vi "rp_change_representation.vi"(6 "Variant in":variant, 7 "Shift Pressed?":bool, 8 "error in (no error)":errorcluster, 10 "QD Combo Box Ref":refnum<vi>, 11 "QD Launch VI Ref":refnum<vi>) -> (0 "error out":errorcluster, 4 "Variant out":variant)   [LabVIEW 2019]
doc: "Change the selected numeric or string control/constant representation, radix and modifiers using the quick drop combo box text formatted as: \"[TYPE[ MODS...]]\"\nTYPE = 'u8', 'u16', 'u32', 'u64', 'i8', 'i16', 'i32', 'i64', 'sgl', 'dbl', 'ext'\nMODS = \n 'd': dec/default\n 'x': hex\n 'b': bin/backslash\n 'r': toggle radix visible\n 'h': hide inc/dec buttons\n 's': show inc/dec buttons\n\nExamples:\nNumeric selected +\"u8 x h\" = Unsigned 8-bit representation, display radix as hex and hide inc/dec buttons\nString selected + \"b\" = Display radix in backslash\n\nDefault Shortcut - [V]"
uses:
  <vilib>/numeric/LVNumericRepresentation.ctl
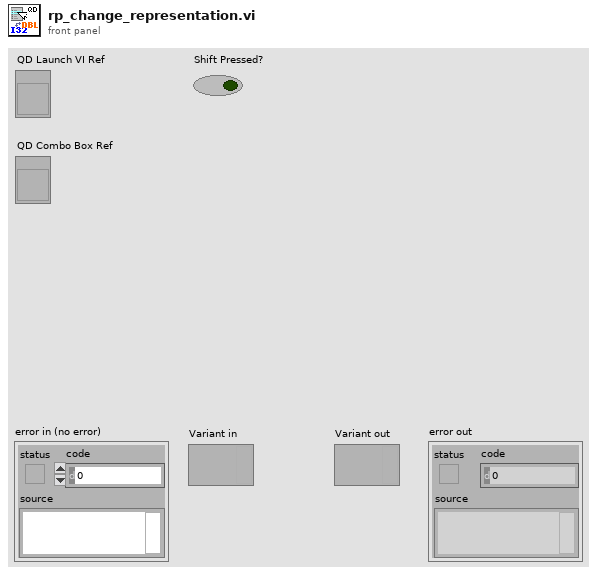
[diagram p1: front panel]
types:
  T1 = typedef "LVNumericRepresentation.ctl" = enum32{"Extended Precision", "Double Precision", "Single Precision", "Long", "Word", "Byte", "Unsigned Long", "Unsigned Word", "Unsigned Byte", "Complex Extended", "Complex Double", "Complex Single", "Quad", "Unsigned Quad", "Fixed-Point"}
  T2 = enum8{"none", "toggle", "decimal", "hex", "binary"}
  T3 = cluster{"DigitalCst":refnum<vi>[], "EnumCst":refnum<vi>[], "RingCst":refnum<vi>[], "StringCst":refnum<vi>[], "Digitals":refnum<vi>[], "Enums":refnum<vi>[], "Rings":refnum<vi>[], "Strings":refnum<vi>[]}
  T4 = typedef "LVRectTypeDef.ctl" = cluster{"Left":i16, "Top":i16, "Right":i16, "Bottom":i16}
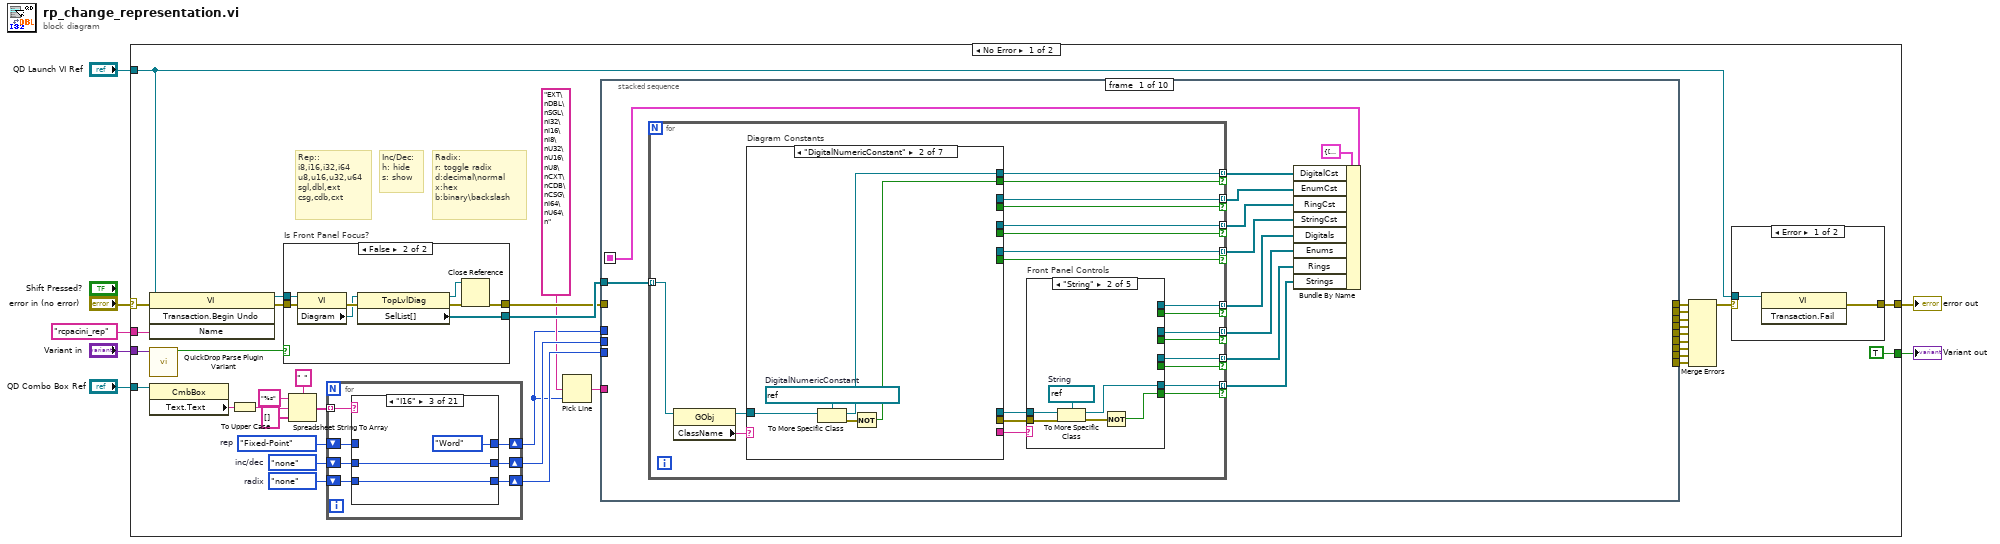
[diagram p0: block diagram]
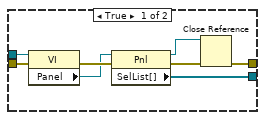
[diagram p2: hidden frame]
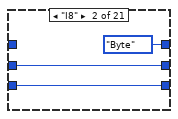
[diagram p4: hidden frame]
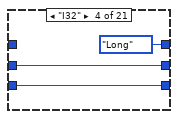
[diagram p5: hidden frame]
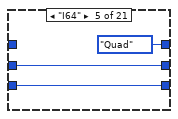
[diagram p6: hidden frame]
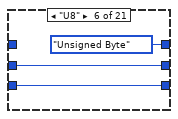
[diagram p7: hidden frame]
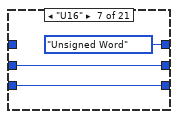
[diagram p8: hidden frame]
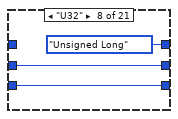
[diagram p9: hidden frame]
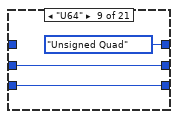
[diagram p10: hidden frame]
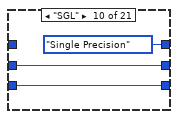
[diagram p11: hidden frame]
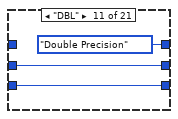
[diagram p12: hidden frame]
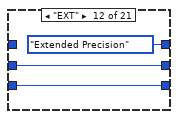
[diagram p13: hidden frame]
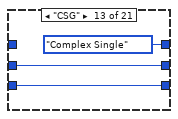
[diagram p14: hidden frame]
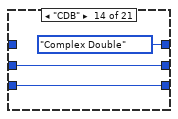
[diagram p15: hidden frame]
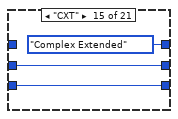
[diagram p16: hidden frame]
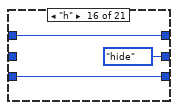
[diagram p17: hidden frame]
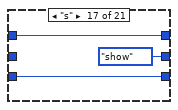
[diagram p18: hidden frame]
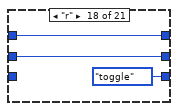
[diagram p19: hidden frame]
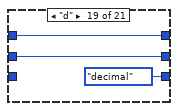
[diagram p20: hidden frame]
diagram:
  n1 = case shown="No Error" "error in (no error)" {
    selector: "error in (no error)" -> [w43 w671]
    tunnel: [w42 w671] -> w1
    tunnel: "QD Launch VI Ref" -> [w36 _]
    tunnel: "rcpacini_rep" ("Undo Name") -> [w41 _]
    tunnel: "Variant in" -> [w9 _]
    tunnel: "QD Combo Box Ref" -> [w37 _]
    tunnel: [TRUE _] -> w2
    frame No Error {
      w26 = enum8{"none", "show", "hide"}."none"  # inc/dec
      w27 = T2."none"  # radix
      w28 = LVNumericRepresentation."Fixed-Point"  # rep
      # "Radix:\nr: toggle radix\nd:decimal\\normal\nx:hex\nb:binary\\backslash"
      # "Inc/Dec:\nh: hide\ns: show"
      # "Rep::\ni8,i16,i32,i64\nu8,u16,u32,u64\nsgl,dbl,ext\ncsg,cdb,cxt"
      n2 = invoke class="VI" method="Transaction.Begin Undo"(reference=w36, error in=w43, "Name"=w41) -> (reference out=w39:refnum<vi>, error out=w40:errorcluster)  [unwired: 1 in, 2 out]
      n3 = call <vilib>:"QuickDrop Parse Plugin Variant.vi"("QDKS Variant in"=w9) -> ("QD Launch VI Panel?"=w8:bool)  [unwired: 12 in, 2 out]
      n4 = property class="CmbBox"(reference=w37) -> ("Text.Text"=w35:string)  [unwired: 1 in, 2 out]
      n5 = To Upper Case(1:w35) -> (0:w34:string)
      n6 = case "Is Front Panel Focus?" shown="False" w8 {
        tunnel: w40 -> [w51 w59]
        tunnel: w39 -> [w50 w58]
        tunnel: [w45 w53] -> w25
        tunnel: [w44 w52] -> w30
        frame True {
          n7 = property class="VI"(reference=w50, error in=w51) -> (error out=w49:errorcluster, "Panel"=w48:refnum<vi>)  [unwired: 1 out]
          n8 = property class="Pnl"(reference=w48, error in=w49) -> (reference out=w46:refnum<vi>, error out=w47:errorcluster, "SelList[]"=w44:refnum<vi>[])
          n9 = Close Reference(reference=w46, error in (no error)=w47) -> (error out=w45:errorcluster)
        }
        frame False {
          n10 = property class="VI"(reference=w58, error in=w59) -> (error out=w57:errorcluster, "Diagram"=w56:refnum<vi>)  [unwired: 1 out]
          n11 = property class="TopLvlDiag"(reference=w56, error in=w57) -> (reference out=w54:refnum<vi>, error out=w55:errorcluster, "SelList[]"=w52:refnum<vi>[])
          n12 = Close Reference(reference=w54, error in (no error)=w55) -> (error out=w53:errorcluster)
        }
      }
      n13 = Spreadsheet String To Array(delimiter (Tab)=" ", format string="%s", spreadsheet string=w34, array type (2D Dbl)=string[] []) -> (array=w29:string[])
      n14 = for {
        tunnel: w29 -> [w66] mode=indexing
        shift-right: [w64] -> w11
        shift-left: w28 -> [w65]
        shift-right: [w63] -> w23
        shift-left: w26 -> [w62]
        shift-right: [w60] -> w22
        shift-left: w27 -> [w61]
        n15 = case shown="\"I16\"" w66 {
          tunnel: w65 -> [w69 _ _ _ _ _ _ _ _ _ _ _ _ _ _ w114 w117 w120 w123 w126 w129]
          tunnel: [w69 LVNumericRepresentation."Byte" ("Representation") LVNumericRepresentation."Word" ("Representation") LVNumericRepresentation."Long" ("Representation") LVNumericRepresentation."Quad" ("Representation") LVNumericRepresentation."Unsigned Byte" ("Representation") LVNumericRepresentation."Unsigned Word" ("Representation") LVNumericRepresentation."Unsigned Long" ("Representation") LVNumericRepresentation."Unsigned Quad" ("Representation") LVNumericRepresentation."Single Precision" ("Representation") LVNumericRepresentation."Double Precision" ("Representation") LVNumericRepresentation."Extended Precision" ("Representation") LVNumericRepresentation."Complex Single" ("Representation") LVNumericRepresentation."Complex Double" ("Representation") LVNumericRepresentation."Complex Extended" ("Representation") w114 w117 w120 w123 w126 w129] -> w64
          tunnel: [w68 w71 w74 w77 w80 w83 w86 w89 w92 w95 w98 w101 w104 w107 w110 enum8{"none", "show", "hide"}."hide" ("inc/dec") enum8{"none", "show", "hide"}."show" ("inc/dec") w119 w122 w125 w128] -> w63
          tunnel: w62 -> [w68 w71 w74 w77 w80 w83 w86 w89 w92 w95 w98 w101 w104 w107 w110 _ _ w119 w122 w125 w128]
          tunnel: [w67 w70 w73 w76 w79 w82 w85 w88 w91 w94 w97 w100 w103 w106 w109 w113 w116 T2."toggle" ("radix") T2."decimal" ("radix") T2."hex" ("radix") T2."binary" ("radix")] -> w60
          tunnel: w61 -> [w67 w70 w73 w76 w79 w82 w85 w88 w91 w94 w97 w100 w103 w106 w109 w113 w116 _ _ _ _]
          frame Default {
          }
          frame "I8" {
          }
          frame "I16" {
          }
          frame "I32" {
          }
          frame "I64" {
          }
          frame "U8" {
          }
          frame "U16" {
          }
          frame "U32" {
          }
          frame "U64" {
          }
          frame "SGL" {
          }
          frame "DBL" {
          }
          frame "EXT" {
          }
          frame "CSG" {
          }
          frame "CDB" {
          }
          frame "CXT" {
          }
          frame "h" {
          }
          frame "s" {
          }
          frame "r" {
          }
          frame "d" {
          }
          frame "x" {
          }
          frame "b" {
          }
        }
      }
      n16 = Pick Line(multi-line string="EXT\nDBL\nSGL\nI32\nI16\nI8\nU32\nU16\nU8\nCXT\nCDB\nCSG\nI64\nU64\n", line index=w11) -> (output string=w10:string)  [unwired: 1 in]
      n17 = stacked-sequence {
        seq-local: [w130 _ _ _ _ _ _ _ _ _] -> [_ w220 w312 w350 w388 w438 w535 w574 w616 _]
        tunnel: w30 -> [w140 _ _ _ _ _ _ _ _ w666]
        tunnel: w25 -> [_ w219 w311 w349 w387 w437 w534 w573 w615 w665]
        tunnel: w11 -> [_ w224 w314 w352 _ w441 w537 w576 _ _]
        tunnel: w23 -> [_ w223 _ _ w389 w440 w536 w575 w617 _]
        tunnel: w22 -> [_ w222 _ _ w390 w439 _ _ w618 _]
        tunnel: [_ w218 _ _ _ _ _ _ _ _] -> w24
        tunnel: w10 -> [_ w221 w313 w351 _ _ _ _ _ _]
        tunnel: [_ _ w310 _ _ _ _ _ _ _] -> w21
        tunnel: [_ _ _ w348 _ _ _ _ _ _] -> w20
        tunnel: [_ _ _ _ w386 _ _ _ _ _] -> w19
        tunnel: [_ _ _ _ _ w436 _ _ _ _] -> w18
        tunnel: [_ _ _ _ _ _ w533 _ _ _] -> w17
        tunnel: [_ _ _ _ _ _ _ w572 _ _] -> w16
        tunnel: [_ _ _ _ _ _ _ _ w614 _] -> w15
        tunnel: [_ _ _ _ _ _ _ _ _ w664] -> w14
        frame #0 {
          n18 = for {
            tunnel: w140 -> [w162] mode=indexing
            tunnel: [w159] -> w139 mode=indexing if=w158
            tunnel: [w157] -> w138 mode=indexing if=w156
            tunnel: [w155] -> w137 mode=indexing if=w154
            tunnel: [w153] -> w136 mode=indexing if=w152
            tunnel: [w148] -> w132 mode=indexing if=w147
            tunnel: [w146] -> w135 mode=indexing if=w145
            tunnel: [w144] -> w134 mode=indexing if=w143
            tunnel: [w142] -> w133 mode=indexing if=w141
            n19 = property class="GObj"(reference=w162) -> (reference out=w160:refnum<vi>, "ClassName"=w161:string)  [unwired: 1 in, 1 out]
            n20 = case "Diagram Constants" shown="\"DigitalNumericConstant\"" w161 {
              selector: w161 -> [_ _ _ _ _ _ w216]
              tunnel: w160 -> [_ w190 w195 w200 w205 w214 w217]
              tunnel: [_ w189 _ _ _ _ _] -> w159
              tunnel: [_ w187 _ _ _ _ _] -> w158
              tunnel: [_ _ w193 _ _ _ _] -> w157
              tunnel: [_ _ w192 _ _ _ _] -> w156
              tunnel: [_ _ _ w198 _ _ _] -> w155
              tunnel: [_ _ _ w197 _ _ _] -> w154
              tunnel: [_ _ _ _ w203 _ _] -> w153
              tunnel: [_ _ _ _ w202 _ _] -> w152
              tunnel: [_ _ _ _ _ w209 w216] -> w149
              tunnel: [_ _ _ _ _ w208 w217] -> w151
              tunnel: [_ _ _ _ _ w207 _] -> w150
              frame Default {
              }
              frame "DigitalNumericConstant" {
                w191 = refnum<vi> refnum  # DigitalNumericConstant
                n21 = To More Specific Class(target class=w191, reference=w190) -> (specific class reference=w189:refnum<vi>, error out=w188:errorcluster)  [unwired: 1 in]
                n22 = Not(x=w188) -> (.not. x?=w187:bool)
              }
              frame "EnumConstant" {
                w196 = refnum<vi> refnum  # EnumConstant
                n23 = To More Specific Class(target class=w196, reference=w195) -> (specific class reference=w193:refnum<vi>, error out=w194:errorcluster)  [unwired: 1 in]
                n24 = Not(x=w194) -> (.not. x?=w192:bool)
              }
              frame "RingConstant" {
                w201 = refnum<vi> refnum  # RingConstant
                n25 = To More Specific Class(target class=w201, reference=w200) -> (specific class reference=w198:refnum<vi>, error out=w199:errorcluster)  [unwired: 1 in]
                n26 = Not(x=w199) -> (.not. x?=w197:bool)
              }
              frame "StringConstant" {
                w206 = refnum<vi> refnum  # StringConstant
                n27 = To More Specific Class(target class=w206, reference=w205) -> (specific class reference=w203:refnum<vi>, error out=w204:errorcluster)  [unwired: 1 in]
                n28 = Not(x=w204) -> (.not. x?=w202:bool)
              }
              frame "ControlTerminal" {
                w215 = refnum<vi> refnum  # ControlTerminal
                n29 = To More Specific Class(target class=w215, reference=w214) -> (specific class reference=w211:refnum<vi>, error out=w213:errorcluster)  [unwired: 1 in]
                n30 = property class="CtrlTerm"(reference=w211, error in=w213) -> (error out=w212:errorcluster, "Control"=w210:refnum<vi>)  [unwired: 1 out]
                n31 = property class="Ctl"(reference=w210, error in=w212) -> (reference out=w208:refnum<vi>, error out=w207:errorcluster, "ClassName"=w209:string)
              }
              frame "Digital", "Enum", "Ring", "String" {
              }
            }
            n32 = case "Front Panel Controls" shown="\"String\"" w149 {
              tunnel: w151 -> [_ w167 w173 w179 w185]
              tunnel: w150 -> [_ w166 w172 w178 w184]
              tunnel: [_ w164 _ _ _] -> w148
              tunnel: [_ w163 _ _ _] -> w147
              tunnel: [_ _ w170 _ _] -> w146
              tunnel: [_ _ w169 _ _] -> w145
              tunnel: [_ _ _ w176 _] -> w144
              tunnel: [_ _ _ w175 _] -> w143
              tunnel: [_ _ _ _ w182] -> w142
              tunnel: [_ _ _ _ w181] -> w141
              frame Default {
              }
              frame "String" {
                w168 = refnum<vi> refnum  # String
                n33 = To More Specific Class(target class=w168, reference=w167, error in=w166) -> (specific class reference=w164:refnum<vi>, error out=w165:errorcluster)
                n34 = Not(x=w165) -> (.not. x?=w163:bool)
              }
              frame "Digital" {
                w174 = refnum<vi> refnum  # Digital
                n35 = To More Specific Class(target class=w174, reference=w173, error in=w172) -> (specific class reference=w170:refnum<vi>, error out=w171:errorcluster)
                n36 = Not(x=w171) -> (.not. x?=w169:bool)
              }
              frame "Enum" {
                w180 = refnum<vi> refnum  # Enum
                n37 = To More Specific Class(target class=w180, reference=w179, error in=w178) -> (specific class reference=w176:refnum<vi>, error out=w177:errorcluster)
                n38 = Not(x=w177) -> (.not. x?=w175:bool)
              }
              frame "Ring" {
                w186 = refnum<vi> refnum  # Ring
                n39 = To More Specific Class(target class=w186, reference=w185, error in=w184) -> (specific class reference=w182:refnum<vi>, error out=w183:errorcluster)
                n40 = Not(x=w183) -> (.not. x?=w181:bool)
              }
            }
          }
          n41 = Bundle By Name(cluster=T3 {"DigitalCst"=[], "EnumCst"=[], "RingCst"=[], "StringCst"=[], "Digitals"=[], "Enums"=[], "Rings"=[], "Strings"=[]} ("refnums"), "DigitalCst"=w139, "EnumCst"=w138, "RingCst"=w137, "StringCst"=w136, "Digitals"=w135, "Enums"=w134, "Rings"=w133, "Strings"=w132) -> (w130:T3)
        }
        frame #1 {
          # "Digital Constants"
          n42 = Unbundle By Name(w220) -> ("DigitalCst"=w225:refnum<vi>[])
          n43 = for {
            tunnel: w225 -> [w238] mode=indexing
            tunnel: w224 -> [w236]
            tunnel: w223 -> [_]
            tunnel: w222 -> [w235]
            tunnel: w219 -> [w237]
            tunnel: w221 -> [w227]
            shift-right: [w229] -> w218
            shift-left: w219 -> [w228]
            n44 = case shown="Default" w236 {
              selector: w236 -> [_ w306]
              tunnel: w238 -> [w302 w309]
              tunnel: w237 -> [w303 w308]
              tunnel: [w303 w307] -> w231
              tunnel: [w302 w305] -> w230
              tunnel: [_ w304] -> w226
              tunnel: w227 -> [_ w304]
              frame "Fixed-Point" {
              }
              frame Default {
                n45 = property class="DigCnst"(reference=w309, error in=w308, "Representation"=w306) -> (reference out=w305:refnum<vi>, error out=w307:errorcluster)
              }
            }
            n46 = case shown="\"decimal\"" w235 {
              tunnel: w231 -> [w254 w260 w271 w285 w301]
              tunnel: w230 -> [w253 w258 w269 w283 w300]
              tunnel: [w254 w262 w273 w287 w296] -> w234
              tunnel: [w253 w261 w272 w286 w294] -> w232
              frame "none" {
              }
              frame "decimal" {
                n47 = property class="DigCnst"(reference=w258, error in=w260) -> (reference out=w257:refnum<vi>, error out=w259:errorcluster, "Representation"=w256:T1)
                n48 = case shown="\"Long\"..\"Unsigned Byte\", \"Quad\", \"Unsigned Quad\"" w256 {
                  tunnel: [_ "%d" "%#_13g"] -> w255
                  frame "Fixed-Point" {
                  }
                  frame "Long".."Unsigned Byte", "Quad", "Unsigned Quad" {
                  }
                  frame "Extended Precision".."Single Precision", "Complex Extended".."Complex Single" {
                  }
                }
                n49 = property class="DigCnst"(reference=w257, error in=w259, "RadixVis"=TRUE ("Radix Visible?"), "FormatString"=w255) -> (reference out=w261:refnum<vi>, error out=w262:errorcluster)
              }
              frame "hex" {
                n50 = property class="DigCnst"(reference=w269, error in=w271) -> (reference out=w268:refnum<vi>, error out=w270:errorcluster, "Representation"=w267:T1)
                n51 = case shown="\"Extended Precision\"..\"Single Precision\", \"Complex Extended\"..\"Complex Single\"" w267 {
                  tunnel: [_ "%02x" "%04x" "%08x" "%016x" "%#_13g"] -> w266
                  frame "Fixed-Point" {
                  }
                  frame "Byte", "Unsigned Byte" {
                  }
                  frame "Word", "Unsigned Word" {
                  }
                  frame "Long", "Unsigned Long" {
                  }
                  frame "Quad", "Unsigned Quad" {
                  }
                  frame "Extended Precision".."Single Precision", "Complex Extended".."Complex Single" {
                  }
                }
                n52 = property class="DigCnst"(reference=w268, error in=w270, "RadixVis"=TRUE ("Radix Visible?"), "FormatString"=w266) -> (reference out=w272:refnum<vi>, error out=w273:errorcluster)
              }
              frame "binary" {
                n53 = property class="DigCnst"(reference=w283, error in=w285) -> (reference out=w282:refnum<vi>, error out=w284:errorcluster, "Representation"=w280:T1)
                n54 = case shown="\"Byte\", \"Unsigned Byte\"" w280 {
                  tunnel: [_ "%08b" "%016b" "%032b" "%064b" "%#_13g"] -> w281
                  frame "Fixed-Point" {
                  }
                  frame "Byte", "Unsigned Byte" {
                  }
                  frame "Word", "Unsigned Word" {
                  }
                  frame "Long", "Unsigned Long" {
                  }
                  frame "Quad", "Unsigned Quad" {
                  }
                  frame "Extended Precision".."Single Precision", "Complex Extended".."Complex Single" {
                  }
                }
                n55 = property class="DigCnst"(reference=w282, error in=w284, "RadixVis"=TRUE ("Radix Visible?"), "FormatString"=w281) -> (reference out=w286:refnum<vi>, error out=w287:errorcluster)
              }
              frame "toggle" {
                n56 = property class="DigCnst"(reference=w300, error in=w301) -> (reference out=w298:refnum<vi>, error out=w299:errorcluster, "RadixVis"=w297:bool)
                n57 = Not(x=w297) -> (.not. x?=w295:bool)
                n58 = property class="DigCnst"(reference=w298, error in=w299, "RadixVis"=w295) -> (reference out=w294:refnum<vi>, error out=w296:errorcluster)
              }
            }
            n59 = case shown="Default" w226 {
              selector: w226 -> [_ w249]
              tunnel: w234 -> [w239 w252]
              tunnel: [w239 w241] -> w233
              tunnel: w232 -> [_ w251]
              frame "" {
              }
              frame Default {
                n60 = property class="DigCnst"(reference=w251, error in=w252, "Label.Visible"=TRUE, "Label.Text"=w249) -> (reference out=w247:refnum<vi>, error out=w248:errorcluster)
                n61 = property class="DigCnst"(reference=w247, error in=w248) -> (error out=w240:errorcluster, "Label"=w246:refnum<vi>, "MasterRect"=w244:T4)  [unwired: 1 out]
                n62 = call "rp_move_label.vi"("error in (no error)"=w240, "Master Bounds Rect"=w244, "Is Source? (F)"=TRUE, "Label in"=w246) -> ("error out"=w242:errorcluster, "dup Label"=w243:refnum<vi>)  [unwired: 6 in]
                n63 = Close Reference(reference=w243, error in (no error)=w242) -> (error out=w241:errorcluster)
              }
            }
            n64 = Merge Errors(w228, w233) -> (w229:errorcluster)
          }
        }
        frame #2 {
          # "Enum Constants"
          n65 = Unbundle By Name(w312) -> ("EnumCst"=w315:refnum<vi>[])
          n66 = for {
            tunnel: w315 -> [w325] mode=indexing
            tunnel: w314 -> [w323]
            tunnel: w311 -> [w324]
            tunnel: w313 -> [w316]
            shift-right: [w319] -> w310
            shift-left: w311 -> [w318]
            n67 = case shown="\"Unsigned Long\"..\"Unsigned Byte\"" w323 {
              selector: w323 -> [_ w344]
              tunnel: w325 -> [w340 w347]
              tunnel: w324 -> [w341 w346]
              tunnel: [w341 w345] -> w322
              tunnel: [w340 w343] -> w321
              tunnel: [_ w342] -> w317
              tunnel: w316 -> [_ w342]
              frame Default {
              }
              frame "Unsigned Long".."Unsigned Byte" {
                n68 = property class="EnmCnst"(reference=w347, error in=w346, "Representation"=w344) -> (reference out=w343:refnum<vi>, error out=w345:errorcluster)
              }
            }
            n69 = case shown="Default" w317 {
              selector: w317 -> [_ w336]
              tunnel: w322 -> [w326 w339]
              tunnel: [w326 w327] -> w320
              tunnel: w321 -> [_ w338]
              frame "" {
              }
              frame Default {
                n70 = property class="EnmCnst"(reference=w338, error in=w339, "Label.Visible"=TRUE, "Label.Text"=w336) -> (reference out=w328:refnum<vi>, error out=w329:errorcluster)
                n71 = property class="EnmCnst"(reference=w328, error in=w329) -> (error out=w330:errorcluster, "Label"=w335:refnum<vi>, "MasterRect"=w333:T4)  [unwired: 1 out]
                n72 = call "rp_move_label.vi"("error in (no error)"=w330, "Master Bounds Rect"=w333, "Is Source? (F)"=TRUE, "Label in"=w335) -> ("error out"=w331:errorcluster, "dup Label"=w332:refnum<vi>)  [unwired: 6 in]
                n73 = Close Reference(reference=w332, error in (no error)=w331) -> (error out=w327:errorcluster)
              }
            }
            n74 = Merge Errors(w318, w320) -> (w319:errorcluster)
          }
        }
        frame #3 {
          # "Ring Constants"
          n75 = Unbundle By Name(w350) -> ("RingCst"=w353:refnum<vi>[])
          n76 = for {
            tunnel: w353 -> [w363] mode=indexing
            tunnel: w352 -> [w361]
            tunnel: w349 -> [w362]
            tunnel: w351 -> [w355]
            shift-right: [w357] -> w348
            shift-left: w349 -> [w356]
            n77 = case shown="Default" w361 {
              selector: w361 -> [_ w382]
              tunnel: w363 -> [w378 w385]
              tunnel: w362 -> [w379 w384]
              tunnel: [w379 w383] -> w360
              tunnel: [w378 w381] -> w358
              tunnel: w355 -> [_ w380]
              tunnel: [_ w380] -> w354
              frame "Complex Extended".."Complex Single", "Fixed-Point" {
              }
              frame Default {
                n78 = property class="RngCnst"(reference=w385, error in=w384, "Representation"=w382) -> (reference out=w381:refnum<vi>, error out=w383:errorcluster)
              }
            }
            n79 = case shown="Default" w354 {
              selector: w354 -> [_ w374]
              tunnel: w360 -> [w364 w377]
              tunnel: [w364 w365] -> w359
              tunnel: w358 -> [_ w376]
              frame "" {
              }
              frame Default {
                n80 = property class="RngCnst"(reference=w376, error in=w377, "Label.Visible"=TRUE, "Label.Text"=w374) -> (reference out=w366:refnum<vi>, error out=w367:errorcluster)
                n81 = property class="RngCnst"(reference=w366, error in=w367) -> (error out=w368:errorcluster, "Label"=w373:refnum<vi>, "MasterRect"=w371:T4)  [unwired: 1 out]
                n82 = call "rp_move_label.vi"("error in (no error)"=w368, "Master Bounds Rect"=w371, "Is Source? (F)"=TRUE, "Label in"=w373) -> ("error out"=w369:errorcluster, "dup Label"=w370:refnum<vi>)  [unwired: 6 in]
                n83 = Close Reference(reference=w370, error in (no error)=w369) -> (error out=w365:errorcluster)
              }
            }
            n84 = Merge Errors(w356, w359) -> (w357:errorcluster)
          }
        }
        frame #4 {
          # "String Constants"
          n85 = Unbundle By Name(w388) -> ("StringCst"=w391:refnum<vi>[])
          n86 = for {
            tunnel: w391 -> [w396] mode=indexing
            tunnel: w390 -> [w399]
            tunnel: w387 -> [w398]
            tunnel: w389 -> [w394]
            shift-right: [w393] -> w386
            shift-left: w387 -> [w392]
            n87 = case shown="\"hide\"" w394 {
              tunnel: w398 -> [w401 w407 w412]
              tunnel: [w401 w406 w411] -> w397
              tunnel: w396 -> [w402 w405 w410]
              tunnel: [w402 w404 w409] -> w395
              frame "none" {
              }
              frame "show" {
                n88 = property class="StrCnst"(reference=w405, error in=w407, "ScrollVis"=TRUE ("Scrollbar Visible?")) -> (reference out=w404:refnum<vi>, error out=w406:errorcluster)
              }
              frame "hide" {
                n89 = property class="StrCnst"(reference=w410, error in=w412, "ScrollVis"=FALSE ("Scrollbar Visible?")) -> (reference out=w409:refnum<vi>, error out=w411:errorcluster)
              }
            }
            n90 = case shown="\"none\"" w399 {
              tunnel: w395 -> [_ w420 w423 w428 w433]
              tunnel: w397 -> [w413 w419 w424 w429 w434]
              tunnel: [w413 w414 w425 w430 w435] -> w400
              frame "none" {
              }
              frame "toggle" {
                n91 = property class="StrCnst"(reference=w420, error in=w419) -> (reference out=w417:refnum<vi>, error out=w418:errorcluster, "DisplayFormatVisibility"=w416:bool)
                n92 = Not(x=w416) -> (.not. x?=w415:bool)
                n93 = property class="StrCnst"(reference=w417, error in=w418, "DisplayFormatVisibility"=w415) -> (error out=w414:errorcluster)  [unwired: 1 out]
              }
              frame "decimal" {
                w421 = u32 0  # normal
                n94 = property class="StrCnst"(reference=w423, error in=w424, "DisplayFormatVisibility"=TRUE ("Display Format Visible?"), "DispStyle"=w421) -> (error out=w425:errorcluster)  [unwired: 1 out]
              }
              frame "hex" {
                w426 = u32 3  # hex
                n95 = property class="StrCnst"(reference=w428, error in=w429, "DisplayFormatVisibility"=TRUE ("Display Format Visible?"), "DispStyle"=w426) -> (error out=w430:errorcluster)  [unwired: 1 out]
              }
              frame "binary" {
                w431 = u32 1  # backslash
                n96 = property class="StrCnst"(reference=w433, error in=w434, "DisplayFormatVisibility"=TRUE ("Display Format Visible?"), "DispStyle"=w431) -> (error out=w435:errorcluster)  [unwired: 1 out]
              }
            }
            n97 = Merge Errors(w392, w400) -> (w393:errorcluster)
          }
        }
        frame #5 {
          # "Digitals"
          n98 = Unbundle By Name(w438) -> ("Digitals"=w442:refnum<vi>[])
          n99 = for {
            tunnel: w442 -> [w457] mode=indexing
            tunnel: w441 -> [w455]
            tunnel: w440 -> [w453]
            tunnel: w439 -> [w450]
            tunnel: w437 -> [w456]
            shift-right: [w448] -> w436
            shift-left: w437 -> [w447]
            n100 = case shown="Default" w455 {
              selector: w455 -> [_ w529]
              tunnel: w457 -> [w526 w532]
              tunnel: w456 -> [w527 w531]
              tunnel: [w527 w530] -> w445
              tunnel: [w526 w528] -> w454
              frame "Fixed-Point" {
              }
              frame Default {
                n101 = property class="DigNum"(reference=w532, error in=w531, "Rep"=w529) -> (reference out=w528:refnum<vi>, error out=w530:errorcluster)
              }
            }
            n102 = property class="DigNum"(reference=w454, error in=w445) -> (reference out=w446:refnum<vi>, error out=w444:errorcluster, "Indicator"=w443:bool)
            n103 = case shown="False" w443 {
              tunnel: w453 -> [w462 _]
              tunnel: [w461 w475] -> w452
              tunnel: [w460 w476] -> w451
              tunnel: w446 -> [w459 w476]
              tunnel: w444 -> [w458 w475]
              frame False {
                n104 = case shown="\"hide\"" w462 {
                  tunnel: w458 -> [w464 w469 w474]
                  tunnel: w459 -> [w463 w468 w473]
                  tunnel: [w464 w466 w471] -> w461
                  tunnel: [w463 w465 w470] -> w460
                  frame "none" {
                  }
                  frame "show" {
                    n105 = property class="DigNum"(reference=w468, error in=w469, "IncDecVis"=TRUE ("Increment/Decrement Visible?")) -> (reference out=w465:refnum<vi>, error out=w466:errorcluster)
                  }
                  frame "hide" {
                    n106 = property class="DigNum"(reference=w473, error in=w474, "IncDecVis"=FALSE ("Increment/Decrement Visible?")) -> (reference out=w470:refnum<vi>, error out=w471:errorcluster)
                  }
                }
              }
              frame True {
              }
            }
            n107 = case shown="\"binary\"" w450 {
              tunnel: w452 -> [w478 w484 w495 w509 w525]
              tunnel: w451 -> [w477 w482 w493 w507 w524]
              tunnel: [w478 w486 w497 w511 w520] -> w449
              tunnel: [w477 w485 w496 w510 w518] -> _
              frame "none" {
              }
              frame "decimal" {
                n108 = property class="DigNum"(reference=w482, error in=w484) -> (reference out=w481:refnum<vi>, error out=w483:errorcluster, "Rep"=w480:T1)
                n109 = case shown="\"Long\"..\"Unsigned Byte\", \"Quad\", \"Unsigned Quad\"" w480 {
                  tunnel: [_ "%d" "%#_13g"] -> w479
                  frame "Fixed-Point" {
                  }
                  frame "Long".."Unsigned Byte", "Quad", "Unsigned Quad" {
                  }
                  frame "Extended Precision".."Single Precision", "Complex Extended".."Complex Single" {
                  }
                }
                n110 = property class="DigNum"(reference=w481, error in=w483, "RadixVis"=TRUE ("Radix Visible?"), "FormatString"=w479) -> (reference out=w485:refnum<vi>, error out=w486:errorcluster)
              }
              frame "hex" {
                n111 = property class="DigNum"(reference=w493, error in=w495) -> (reference out=w492:refnum<vi>, error out=w494:errorcluster, "Rep"=w491:T1)
                n112 = case shown="\"Extended Precision\"..\"Single Precision\", \"Complex Extended\"..\"Complex Single\"" w491 {
                  tunnel: [_ "%02x" "%04x" "%08x" "%016x" "%#_13g"] -> w490
                  frame "Fixed-Point" {
                  }
                  frame "Byte", "Unsigned Byte" {
                  }
                  frame "Word", "Unsigned Word" {
                  }
                  frame "Long", "Unsigned Long" {
                  }
                  frame "Quad", "Unsigned Quad" {
                  }
                  frame "Extended Precision".."Single Precision", "Complex Extended".."Complex Single" {
                  }
                }
                n113 = property class="DigNum"(reference=w492, error in=w494, "RadixVis"=TRUE ("Radix Visible?"), "FormatString"=w490) -> (reference out=w496:refnum<vi>, error out=w497:errorcluster)
              }
              frame "binary" {
                n114 = property class="DigNum"(reference=w507, error in=w509) -> (reference out=w506:refnum<vi>, error out=w508:errorcluster, "Rep"=w504:T1)
                n115 = case shown="\"Quad\", \"Unsigned Quad\"" w504 {
                  tunnel: [_ "%08b" "%016b" "%032b" "%064b" "%#_13g"] -> w505
                  frame "Fixed-Point" {
                  }
                  frame "Byte", "Unsigned Byte" {
                  }
                  frame "Word", "Unsigned Word" {
                  }
                  frame "Long", "Unsigned Long" {
                  }
                  frame "Quad", "Unsigned Quad" {
                  }
                  frame "Extended Precision".."Single Precision", "Complex Extended".."Complex Single" {
                  }
                }
                n116 = property class="DigNum"(reference=w506, error in=w508, "RadixVis"=TRUE ("Radix Visible?"), "FormatString"=w505) -> (reference out=w510:refnum<vi>, error out=w511:errorcluster)
              }
              frame "toggle" {
                n117 = property class="DigNum"(reference=w524, error in=w525) -> (reference out=w522:refnum<vi>, error out=w523:errorcluster, "RadixVis"=w521:bool)
                n118 = Not(x=w521) -> (.not. x?=w519:bool)
                n119 = property class="DigNum"(reference=w522, error in=w523, "RadixVis"=w519) -> (reference out=w518:refnum<vi>, error out=w520:errorcluster)
              }
            }
            n120 = Merge Errors(w447, w449) -> (w448:errorcluster)
          }
        }
        frame #6 {
          # "Enums"
          n121 = Unbundle By Name(w535) -> ("Enums"=w538:refnum<vi>[])
          n122 = for {
            tunnel: w538 -> [w550] mode=indexing
            tunnel: w537 -> [w548]
            tunnel: w534 -> [w549]
            tunnel: w536 -> [w545]
            shift-right: [w544] -> w533
            shift-left: w534 -> [w543]
            n123 = case shown="\"Unsigned Long\"..\"Unsigned Byte\"" w548 {
              selector: w548 -> [_ w568]
              tunnel: w550 -> [w565 w571]
              tunnel: w549 -> [w566 w570]
              tunnel: [w566 w569] -> w541
              tunnel: [w565 w567] -> w546
              frame Default {
              }
              frame "Unsigned Long".."Unsigned Byte" {
                n124 = property class="Enum"(reference=w571, error in=w570, "Rep"=w568) -> (reference out=w567:refnum<vi>, error out=w569:errorcluster)
              }
            }
            n125 = property class="Enum"(reference=w546, error in=w541) -> (reference out=w542:refnum<vi>, error out=w540:errorcluster, "Indicator"=w539:bool)
            n126 = case shown="False" w539 {
              tunnel: w540 -> [w554 w564]
              tunnel: [w553 w564] -> w547
              tunnel: w542 -> [w552 _]
              tunnel: w545 -> [w551 _]
              frame False {
                n127 = case shown="\"hide\"" w551 {
                  tunnel: w554 -> [w555 w559 w563]
                  tunnel: w552 -> [_ w558 w562]
                  tunnel: [w555 w556 w560] -> w553
                  frame "none" {
                  }
                  frame "show" {
                    n128 = property class="Enum"(reference=w558, error in=w559, "IncDecVis"=TRUE ("Increment/Decrement Visible?")) -> (error out=w556:errorcluster)  [unwired: 1 out]
                  }
                  frame "hide" {
                    n129 = property class="Enum"(reference=w562, error in=w563, "IncDecVis"=FALSE ("Increment/Decrement Visible?")) -> (error out=w560:errorcluster)  [unwired: 1 out]
                  }
                }
              }
              frame True {
              }
            }
            n130 = Merge Errors(w543, w547) -> (w544:errorcluster)
          }
        }
        frame #7 {
          # "Rings"
          n131 = Unbundle By Name(w574) -> ("Rings"=w577:refnum<vi>[])
          n132 = for {
            tunnel: w577 -> [w589] mode=indexing
            tunnel: w576 -> [w587]
            tunnel: w573 -> [w588]
            tunnel: w575 -> [w584]
            shift-right: [w583] -> w572
            shift-left: w573 -> [w582]
            n133 = case shown="Default" w587 {
              selector: w587 -> [_ w610]
              tunnel: w589 -> [w607 w613]
              tunnel: w588 -> [w608 w612]
              tunnel: [w608 w611] -> w580
              tunnel: [w607 w609] -> w585
              frame "Complex Extended".."Complex Single", "Fixed-Point" {
              }
              frame Default {
                n134 = property class="Ring"(reference=w613, error in=w612, "Rep"=w610) -> (reference out=w609:refnum<vi>, error out=w611:errorcluster)
              }
            }
            n135 = property class="Ring"(reference=w585, error in=w580) -> (reference out=w581:refnum<vi>, error out=w579:errorcluster, "Indicator"=w578:bool)
            n136 = case shown="False" w578 {
              tunnel: w579 -> [w593 w606]
              tunnel: [w592 w606] -> w586
              tunnel: w581 -> [w591 _]
              tunnel: w584 -> [w590 _]
              frame False {
                n137 = case shown="\"hide\"" w590 {
                  tunnel: w593 -> [w595 w600 w605]
                  tunnel: w591 -> [w594 w599 w604]
                  tunnel: [w595 w597 w602] -> w592
                  tunnel: [w594 w596 w601] -> _
                  frame "none" {
                  }
                  frame "show" {
                    n138 = property class="Ring"(reference=w599, error in=w600, "IncDecVis"=TRUE ("Increment/Decrement Visible?")) -> (reference out=w596:refnum<vi>, error out=w597:errorcluster)
                  }
                  frame "hide" {
                    n139 = property class="Ring"(reference=w604, error in=w605, "IncDecVis"=FALSE ("Increment/Decrement Visible?")) -> (reference out=w601:refnum<vi>, error out=w602:errorcluster)
                  }
                }
              }
              frame True {
              }
            }
            n140 = Merge Errors(w582, w586) -> (w583:errorcluster)
          }
        }
        frame #8 {
          # "Strings"
          n141 = Unbundle By Name(w616) -> ("Strings"=w619:refnum<vi>[])
          n142 = for {
            tunnel: w619 -> [w625] mode=indexing
            tunnel: w618 -> [w627]
            tunnel: w615 -> [w626]
            tunnel: w617 -> [w622]
            shift-right: [w621] -> w614
            shift-left: w615 -> [w620]
            n143 = case shown="\"show\"" w622 {
              tunnel: w626 -> [w629 w635 w640]
              tunnel: [w629 w634 w639] -> w624
              tunnel: w625 -> [w630 w633 w638]
              tunnel: [w630 w632 w637] -> w623
              frame "none" {
              }
              frame "show" {
                n144 = property class="Str"(reference=w633, error in=w635, "VScrollVis"=TRUE ("Scrollbar Visible?")) -> (reference out=w632:refnum<vi>, error out=w634:errorcluster)
              }
              frame "hide" {
                n145 = property class="Str"(reference=w638, error in=w640, "VScrollVis"=FALSE ("Scrollbar Visible?")) -> (reference out=w637:refnum<vi>, error out=w639:errorcluster)
              }
            }
            n146 = case shown="\"hex\"" w627 {
              tunnel: w623 -> [_ w648 w651 w656 w661]
              tunnel: w624 -> [w641 w647 w652 w657 w662]
              tunnel: [w641 w642 w653 w658 w663] -> w628
              frame "none" {
              }
              frame "toggle" {
                n147 = property class="Str"(reference=w648, error in=w647) -> (reference out=w645:refnum<vi>, error out=w646:errorcluster, "DisplayFormatVisibility"=w644:bool)
                n148 = Not(x=w644) -> (.not. x?=w643:bool)
                n149 = property class="Str"(reference=w645, error in=w646, "DisplayFormatVisibility"=w643) -> (error out=w642:errorcluster)  [unwired: 1 out]
              }
              frame "decimal" {
                w649 = u32 0  # normal
                n150 = property class="Str"(reference=w651, error in=w652, "DisplayFormatVisibility"=TRUE ("Display Format Visible?"), "Display Style"=w649) -> (error out=w653:errorcluster)  [unwired: 1 out]
              }
              frame "hex" {
                w654 = u32 3  # hex
                n151 = property class="Str"(reference=w656, error in=w657, "DisplayFormatVisibility"=TRUE ("Display Format Visible?"), "Display Style"=w654) -> (error out=w658:errorcluster)  [unwired: 1 out]
              }
              frame "binary" {
                w659 = u32 1  # backslash
                n152 = property class="Str"(reference=w661, error in=w662, "DisplayFormatVisibility"=TRUE ("Display Format Visible?"), "Display Style"=w659) -> (error out=w663:errorcluster)  [unwired: 1 out]
              }
            }
            n153 = Merge Errors(w620, w628) -> (w621:errorcluster)
          }
        }
        frame #9 {
          n154 = Close Reference(reference=w666, error in (no error)=w665) -> (error out=w664:errorcluster)
        }
      }
      n155 = Merge Errors(w24, w21, w20, w19, w18, w17, w16, w15, w14) -> (w13:errorcluster)
      n156 = case shown="Error" w13 {
        tunnel: w36 -> [w667 w669]
        tunnel: [w668 w670] -> w42
        frame Error {
          n157 = invoke class="VI" method="Transaction.Fail"(reference=w667) -> (error out=w668:errorcluster)  [unwired: 2 in, 2 out]
        }
        frame No Error {
          n158 = invoke class="VI" method="Transaction.End Undo"(reference=w669) -> (error out=w670:errorcluster)  [unwired: 2 in, 2 out]
        }
      }
    }
    frame Error {
    }
  }
  "error out" <- w1
  "Variant out" <- w2
